vi "Get Hi Limit.vi"(8 "error in (no error)":errorcluster, 11 "VISA resource name":refnum<visa-resource-name>) -> (0 "error out":errorcluster, 2 "Hi Limit":dbl, 3 "VISA resource name out":refnum<visa-resource-name>)   [LabVIEW 2012, in "Associated Research 78XX Series.lvlib"]
uses:
  <instrlib>/Associated Research 78XX Series/Associated Research 78XX Series.lvlib
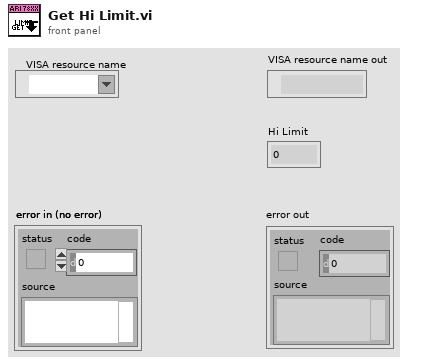
[diagram p1: front panel]
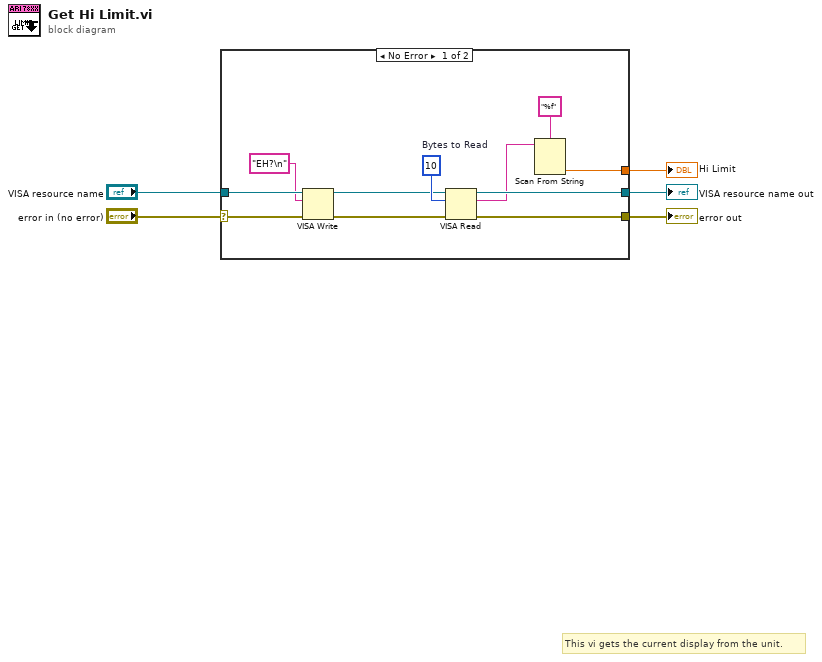
[diagram p0: block diagram]
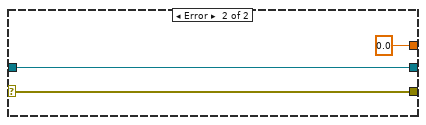
[diagram p2: hidden frame]
diagram:
  # "This vi gets the current display from the unit."
  n1 = case shown="No Error" "error in (no error)" {
    selector: "error in (no error)" -> [w16 w19]
    tunnel: [w12 w19] -> w4
    tunnel: [w8 w18] -> w2
    tunnel: "VISA resource name" -> [w15 w18]
    tunnel: [w6 0.0] -> w1
    frame No Error {
      w14 = u32 10  # Bytes to Read
      n2 = VISA Write(VISA resource name=w15, write buffer="EH?\n" ("string (\"\")"), error in (no error)=w16) -> (VISA resource name out=w11:refnum<visa-resource-name>, error out=w10:errorcluster)  [unwired: 1 out]
      n3 = VISA Read(VISA resource name=w11, byte count=w14, error in (no error)=w10) -> (VISA resource name out=w8:refnum<visa-resource-name>, read buffer=w7:string, error out=w12:errorcluster)  [unwired: 1 out]
      n4 = Scan From String(format string="%f", input string=w7) -> (output 1=w6:dbl)  [unwired: 3 in, 3 out]
    }
    frame Error {
    }
  }
  "error out" <- w4
  "VISA resource name out" <- w2
  "Hi Limit" <- w1
